vi "Replace.vi"(8 "error in (no error)":errorcluster, 11 "CConfig By Ref Buffer in":refnum<class "CConfig By Ref Buffer.lvclass">) -> (0 "error out":errorcluster, 2 "Replace?":bool=TRUE, 3 "CConfig By Ref Buffer out":refnum<class "CConfig By Ref Buffer.lvclass">)   [LabVIEW 2013, in "CConfig By Ref Buffer.lvclass"]
doc: "Copyright 2018, Carya Automatisering, Wiebe Walstra."
uses:
  CConfig By Ref Buffer.lvclass
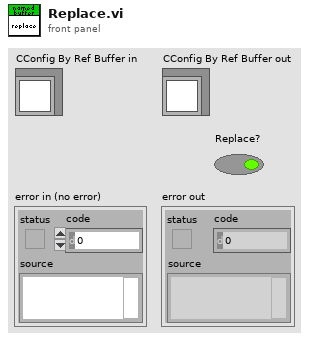
[diagram p1: front panel]
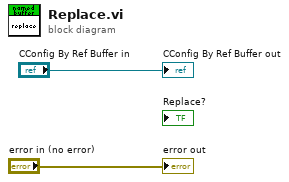
[diagram p0: block diagram]
diagram:
  "error out" <- "error in (no error)"
  "CConfig By Ref Buffer out" <- "CConfig By Ref Buffer in"
